vi "roboRIO v1.0 Reserve DIO.vi"(7 "Allow multiple opens?":bool, 8 "error in (no error)":errorcluster, 10 "DIO Channel List":T2, 11 "myRIO FPGA Ref Out":T1) -> (0 "error out":errorcluster)   [LabVIEW 2021]
uses:
  <vilib>/myRIO/Common/Instrument Driver Framework/myRIO v1.0/DIO/typedefs/DIO Channels List.ctl
  <vilib>/myRIO/Common/Instrument Driver Framework/myRIO v1.0/DIO/typedefs/DIO Channels Enum.ctl
  <vilib>/myRIO/Common/Instrument Driver Framework/Utilities/typedefs/Generic FPGA Reference.ctl
  <vilib>/myRIO/Common/Instrument Driver Framework/roboRIO v1.0/Resource Manager/vis/roboRIO v1.0 Create Configuration List.vi
  <vilib>/myRIO/Common/Instrument Driver Framework/roboRIO v1.0/Resource Manager/vis/roboRIO v1.0 Reserve Channel.vi
  <vilib>/myRIO/Common/Instrument Driver Framework/roboRIO v1.0/Resource Manager/vis/roboRIO v1.0 Unreserve Channel.vi
  <vilib>/myRIO/Common/Instrument Driver Framework/roboRIO v1.0/Resource Manager/vis/roboRIO v1.0 Build Mutex Name.vi
  <vilib>/myRIO/Common/Instrument Driver Framework/Utilities/vis/IO Manager.vi
  <vilib>/Utility/error.llb/Error Cluster From Error Code.vi
  <vilib>/myRIO/Common/Instrument Driver Framework/Utilities/vis/Configuration Manager.vi
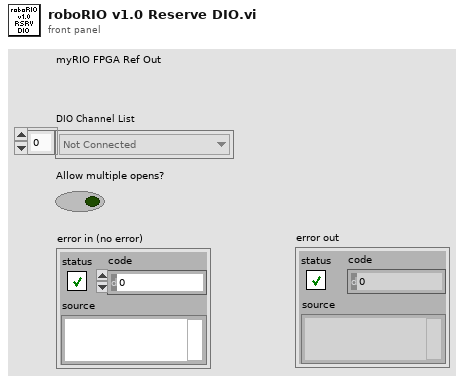
[diagram p1: front panel]
types:
  T1 = typedef "Generic FPGA Reference.ctl" = refnum<k20>
  T2 = typedef "DIO Channels List.ctl" = T3[]
  T3 = typedef "DIO Channels Enum.ctl" = enum16{"Not Connected", "C/DIO0", "C/DIO1", "C/DIO2", "C/DIO3", "C/DIO4", "C/DIO5", "C/DIO6", "C/DIO7", "A/DIO0", "A/DIO1", "A/DIO2", "A/DIO3", "A/DIO4", "A/DIO5", "A/DIO6", "A/DIO7", "A/DIO8", "A/DIO9", "A/DIO10", "A/DIO11", "A/DIO12", "A/DIO13", "A/DIO14", "A/DIO15", "A/DIO16", "A/DIO17", "A/DIO18", "A/DIO19", "B/DIO0", "B/DIO1", "B/DIO2", "B/DIO3", "B/DIO4", "B/DIO5", "B/DIO6", "B/DIO7", "B/DIO8", "B/DIO9", "B/DIO10", "B/DIO11", "B/DIO12", "B/DIO13", "B/DIO14", "B/DIO15", "B/DIO16", "B/DIO17", "B/DIO18", "B/DIO19", "LED0", "LED1", "LED2", "LED3", "Button0", "DIO/DIO0", "DIO/DIO1", "DIO/DIO2", "DIO/DIO3", "DIO/DIO4", "DIO/DIO5", "DIO/DIO6", "DIO/DIO7", "DIO/DIO8", "DIO/DIO9", "SPI/CS0", "SPI/CS1", "SPI/CS2", "SPI/CS3", "LED RADIO (Green)", "LED RADIO (Red)", "LED COMM (Green)", "LED COMM (Red)", "LED MODE (Green)", "LED MODE (Red)"}
  T4 = typedef "roboRIO v1.0 Channel Reservation List.ctl" = T5[]
  T5 = typedef "roboRIO v1.0 Channel Reservation Info.ctl" = cluster{"Channel Name":string, "Connector":T6, "Mutex ID":i32}
  T6 = typedef "roboRIO v1.0 Connector List.ctl" = enum32{"None", "ConnectorB", "ConnectorI2C", "ConnectorDIO", "ConnectorRSL", "ConnectorRELAY", "ConnectorAI", "ConnectorPWM", "ConnectorSPI"}
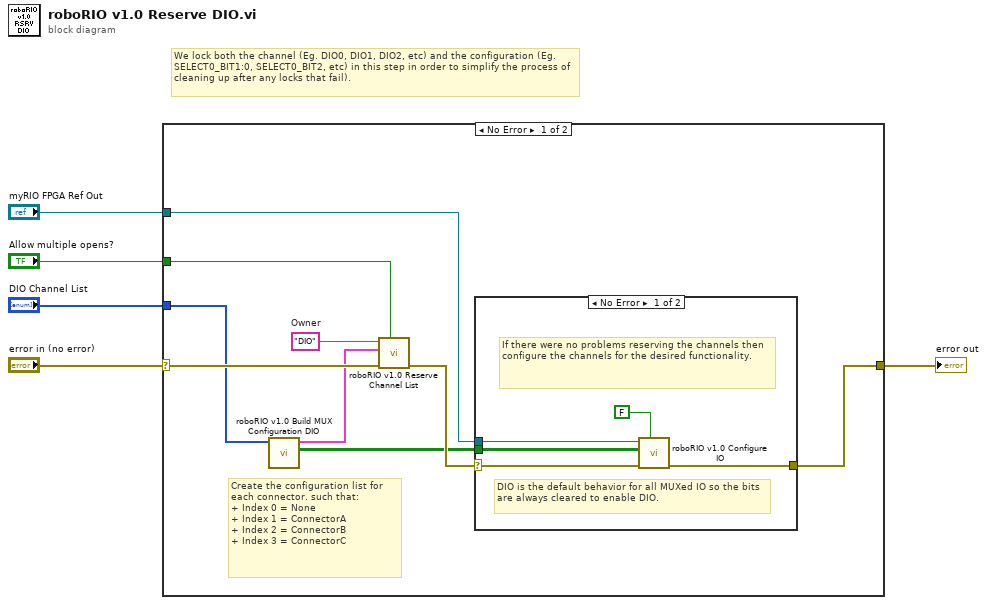
[diagram p0: block diagram]
diagram:
  # "We lock both the channel (Eg. DIO0, DIO1, DIO2, etc) and the configuration (Eg. SELECT0_BIT1:0, SELECT0_BIT2, etc) in this step in order to simplify the process of cleaning up after any locks that fail)."
  n1 = case shown="No Error" "error in (no error)" {
    selector: "error in (no error)" -> [w12 w21]
    tunnel: "myRIO FPGA Ref Out" -> [w11 _]
    tunnel: "DIO Channel List" -> [w6 _]
    tunnel: [w14 w21] -> w3
    tunnel: "Allow multiple opens?" -> [w13 _]
    frame No Error {
      w10 = "DIO"  # Owner
      # "Create the configuration list for each connector. such that:\n+ Index 0 = None\n+ Index 1 = ConnectorA\n+ Index 2 = ConnectorB \n+ Index 3 = ConnectorC"
      n2 = call <vilib>:"roboRIO v1.0 Build MUX Configuration DIO.vi"("DIO Channel List"=w6) -> ("Configuration Bitmask Array"=w7:bool[][], "Channel Reservation List"=w8:T4)  [unwired: 9 in]
      n3 = call <vilib>:"roboRIO v1.0 Reserve Channel List.vi"("Allow multiple opens?"=w13, "error in (no error)"=w12, "Channel Reservation List"=w8, "Owner"=w10) -> ("error out"=w9:errorcluster)  [unwired: 7 in]
      n4 = case shown="No Error" w9 {
        selector: w9 -> [w17 w20]
        tunnel: w11 -> [w19 _]
        tunnel: w7 -> [w16 _]
        tunnel: [w15 w20] -> w14
        frame No Error {
          # "If there were no problems reserving the channels then configure the channels for the desired functionality."
          # "DIO is the default behavior for all MUXed IO so the bits are always cleared to enable DIO."
          n5 = call <vilib>:"roboRIO v1.0 Configure IO.vi"("Value"=FALSE ("Clear?"), "error in (no error)"=w17, "Bitmask Array"=w16, "myRIO FPGA Ref In"=w19) -> ("error out"=w15:errorcluster)  [unwired: 7 in]
        }
        frame Error {
        }
      }
    }
    frame Error {
    }
  }
  "error out" <- w3
